vi "FMTone-Create.vi"(0 "FM":T1, 7 "Sampling Rate (Hz)":dbl, 9 "Npts":i32, 11 "error in (no error)":errorcluster) -> (8 "WF":dbl[](array[numeric]), 15 "error out":errorcluster)   [LabVIEW 2020]
uses:
  XControls/Waveform XControls/FM Tone/Data.ctl
  Utility VIs/Math VIs/LinSpace (x0-dx-npts).vi
  XControls/Waveform XControls/FM Tone/FM Tone.xctl
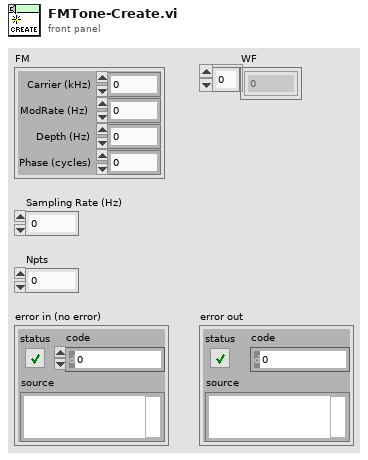
[diagram p1: front panel]
types:
  T1 = typedef "FM Tone.xctl/Data.ctl" = cluster{"Carrier (kHz)":dbl, "ModRate (Hz)":dbl, "Depth (Hz)":dbl, "Phase (cycles)":dbl}
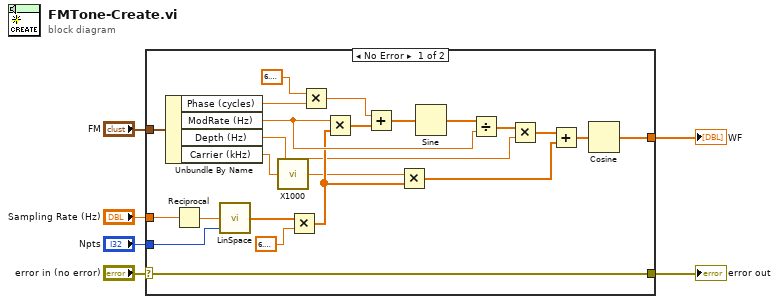
[diagram p0: block diagram]
diagram:
  n1 = case shown="No Error" "error in (no error)" {
    selector: "error in (no error)" -> [w29 w30]
    tunnel: [w29 w30] -> w2
    tunnel: [w7 _] -> w3
    tunnel: "FM" -> [w25 _]
    tunnel: "Sampling Rate (Hz)" -> [w28 _]
    tunnel: "Npts" -> [w26 _]
    frame No Error {
      n2 = Unbundle By Name(w25) -> ("Phase (cycles)"=w20:dbl, "ModRate (Hz)"=w16:dbl, "Depth (Hz)"=w13:dbl, "Carrier (kHz)"=w12:dbl)
      n3 = Reciprocal(x=w28) -> (1/x=w27:dbl)
      n4 = call-poly "LinSpace.vi"("npts"=w26, "dx"=w27) -> ("Array"=w24:dbl[])  [unwired: 2 in, 1 out]
      n5 = call "X1000.vi"("X"=w12) -> ("X/1000"=w11:dbl)
      n6 = Multiply(x=w24, y=6.283185307179586) -> (x*y=w15:dbl[])
      n7 = Multiply(x=6.283185307179586, y=w20) -> (x*y=w19:dbl)
      n8 = Multiply(x=w16, y=w15) -> (x*y=w22:dbl[])
      n9 = Add(x=w19, y=w22) -> (x+y=w18:dbl[])
      n10 = Multiply(x=w11, y=w15) -> (x*y=w9:dbl[])
      n11 = Sine(x=w18) -> (sin(x)=w17:dbl[])
      n12 = Divide(x=w17, y=w16) -> (x/y=w14:dbl[])
      n13 = Multiply(x=w14, y=w13) -> (x*y=w10:dbl[])
      n14 = Add(x=w10, y=w9) -> (x+y=w8:dbl[])
      n15 = Cosine(x=w8) -> (cos(x)=w7:dbl[])
    }
    frame Error {
    }
  }
  "WF" <- w3
  "error out" <- w2
